vi "Calibration-Line1-CalMain.vi"(8 "error in (no error)":errorcluster, 11 "Calibration-RunTest in":refnum<class "Calibration-RunTest.lvclass">) -> (0 "error out":errorcluster, 3 "Calibration-RunTest out":refnum<class "Calibration-RunTest.lvclass">)   [LabVIEW 2013, in "Calibration-RunTest.lvclass"]
uses:
  Calibration-RunTest.lvclass
  Calibration-RunTest.lvclass/Calibration-RunTest.ctl
  Motion Control/Motion-ControlAll.lvclass
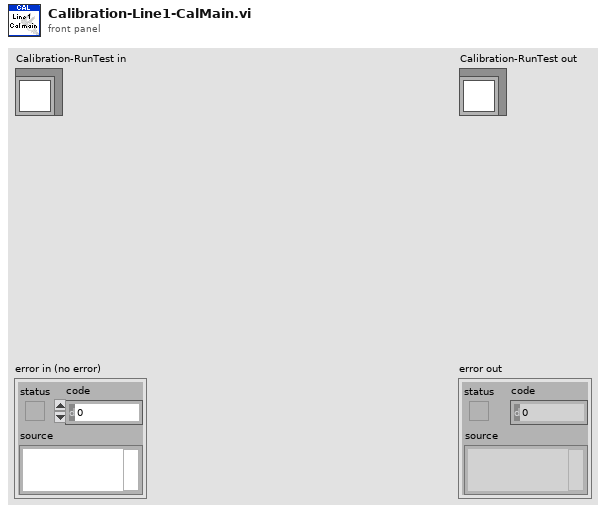
[diagram p1: front panel]
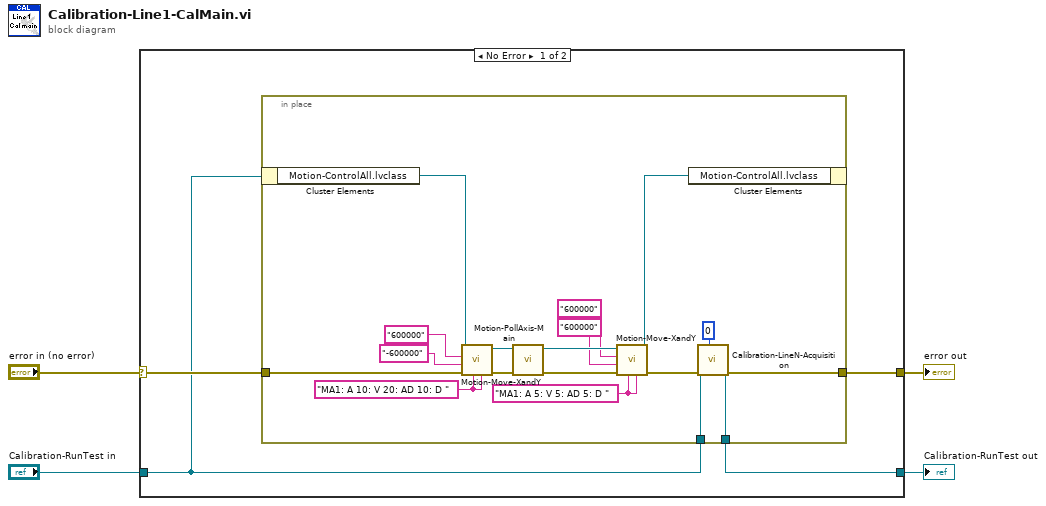
[diagram p0: block diagram]
diagram:
  n1 = case shown="No Error" "error in (no error)" {
    selector: "error in (no error)" -> [w8 w28]
    tunnel: [w7 w28] -> w3
    tunnel: [w5 w27] -> w1
    tunnel: "Calibration-RunTest in" -> [w6 w27]
    frame No Error {
      n2 = in-place {
        in-place-border: w8 -> [w15]
        in-place-border: [w10] -> w7
        in-place-border: w6 -> [w12]
        in-place-border: [w9] -> w5
        w26 = "MA1: A 10: V 20: AD 10: D " ("concatenated string")
        w25 = "MA1: A 5: V 5: AD 5: D " ("concatenated string")
        n3 = in-place-cluster #1(w6) -> ("Motion-ControlAll.lvclass"=w16:refnum<class "Motion-ControlAll.lvclass">)
        n4 = call "Motion-Move-XandY.vi"("Y Drive Acc/Speed/Velocity"=w26, "X Drive Acc/Speed/Velocity"=w26, "error in (no error)"=w15, "X Coordinates"="-600000", "Y Coordinates"="600000", "Motion-ControlAll in"=w16) -> ("error out"=w18:errorcluster, "Motion-ControlAll out"=w17:refnum<class "Motion-ControlAll.lvclass">)  [unwired: 4 in]
        n5 = call "Motion-PollAxis-Main.vi"("error in (no error)"=w18, "Motion-ControlAll in"=w17) -> ("error out"=w23:errorcluster, "Motion-ControlAll out"=w24:refnum<class "Motion-ControlAll.lvclass">)  [unwired: 8 in]
        n6 = call "Motion-Move-XandY.vi"("Y Drive Acc/Speed/Velocity"=w25, "X Drive Acc/Speed/Velocity"=w25, "error in (no error)"=w23, "X Coordinates"="600000", "Y Coordinates"="600000", "Motion-ControlAll in"=w24) -> ("error out"=w14:errorcluster, "Motion-ControlAll out"=w13:refnum<class "Motion-ControlAll.lvclass">)  [unwired: 4 in]
        n7 = in-place-cluster #1("Motion-ControlAll.lvclass"=w13) -> ()  [unwired: 1 out]
        n8 = call "Calibration-LineN-Acquisition.vi"("Cal Line?"=0, "error in (no error)"=w14, "Calibration-RunTest in"=w12) -> ("error out"=w10:errorcluster, "Calibration-RunTest out"=w9:refnum<class "Calibration-RunTest.lvclass">)  [unwired: 7 in]
      }
    }
    frame Error {
    }
  }
  "error out" <- w3
  "Calibration-RunTest out" <- w1
